vi "test 1588 Deployment.vi"(8 "error in (no error)":errorcluster, 11 "TestCase in":refnum<class "Linux x64 System Tests.lvclass">) -> (0 "error out":errorcluster, 3 "TestCase out":refnum<class "Linux x64 System Tests.lvclass">)   [LabVIEW 2015, in "Linux x64 System Tests.lvclass"]
uses:
  Linux x64 System Tests.lvclass
  Shared/Constants.vi
  <vilib>/addons/_JKI Toolkits/VI Tester/TestCase.llb/TestCase.lvclass
  Shared/NI Synchronization Shared.lvlib
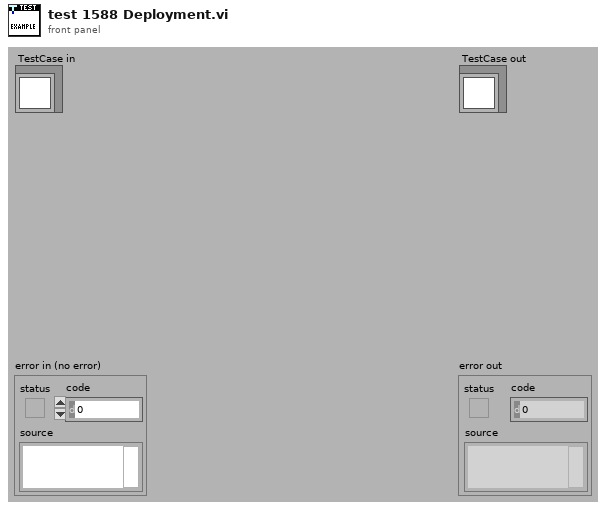
[diagram p1: front panel]
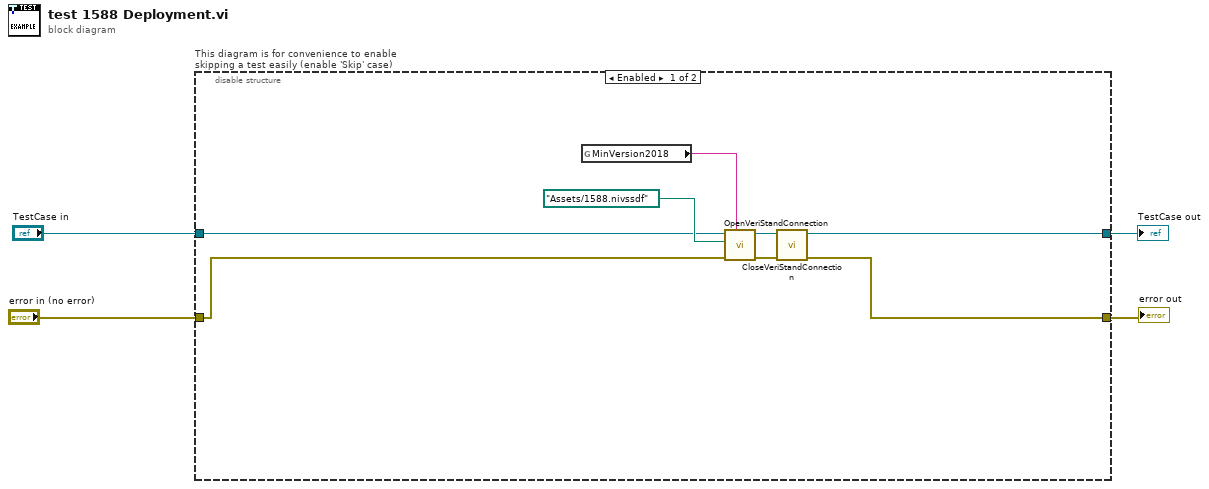
[diagram p0: block diagram]
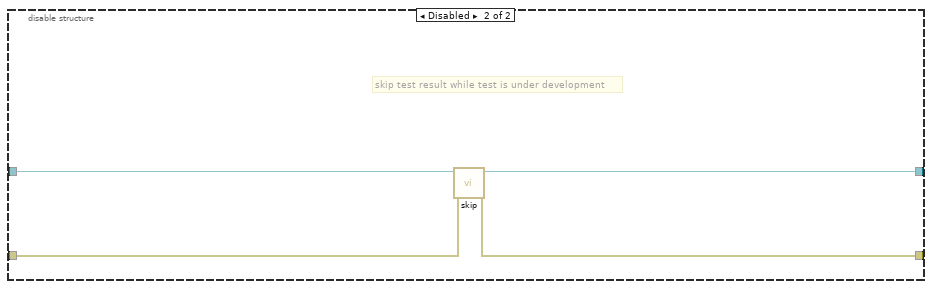
[diagram p2: hidden frame]
diagram:
  n1 = disable-structure "This diagram is for convenience to enable skipping a test easily (enable 'Skip' case)" shown="Enabled" {
    disable-tunnel: "TestCase in" -> [w9 w16]
    disable-tunnel: [w8 w14] -> w1
    disable-tunnel: [w6 w15] -> w3
    disable-tunnel: "error in (no error)" -> [w7 w13]
    frame Enabled {
      n2 = global read "Constants.vi" "MinVersion2018"() -> (w5:string)
      n3 = call-dynamic "OpenVeriStandConnection.vi"("Minimum VeriStand Version (2015)"=w5, "error in (no error)"=w7, "System Definition File"=path "Assets/1588.nivssdf", "VeriStand Test Case in"=w9) -> ("error out"=w11:errorcluster, "VeriStand Test Case out"=w12:refnum<class "Linux x64 System Tests.lvclass">)  [unwired: 5 in, 1 out]
      n4 = call-dynamic "CloseVeriStandConnection.vi"("error in (no error)"=w11, "VeriStand Test Case in"=w12) -> ("error out"=w6:errorcluster, "VeriStand Test Case out"=w8:refnum<class "Linux x64 System Tests.lvclass">)  [unwired: 8 in]
    }
    frame Disabled {
      # "skip test result while test is under development"
      n5 = call <vilib>:"skip.vi"("error in (no error)"=w13, "TestCase in"=w16) -> ("error out"=w15:errorcluster, "TestCase out"=w14:refnum<class "Linux x64 System Tests.lvclass">)  [unwired: 8 in]
    }
  }
  "error out" <- w3
  "TestCase out" <- w1
